vi "SessionName To IniTokenCluster.vi"(11 "trimmed string":string) -> (3 "IniTokenCluster":T1)   [LabVIEW 2012]
uses:
  Def-IniTokenCluster.ctl
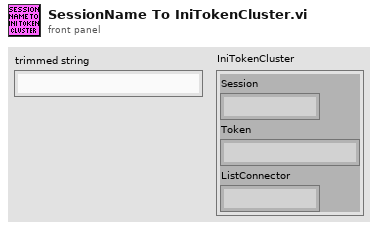
[diagram p1: front panel]
types:
  T1 = typedef "Def-IniTokenCluster.ctl" = cluster{"Session":string, "Token":string, "ListConnector":string}
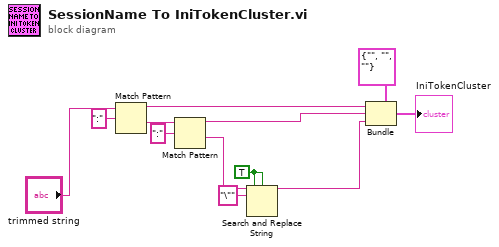
[diagram p0: block diagram]
diagram:
  w9 = TRUE ("ignore case? (F)")
  n1 = Match Pattern(string="trimmed string", regular expression=":") -> (before substring=w4:string, after substring=w1:string)  [unwired: 1 in, 2 out]
  n2 = Match Pattern(string=w1, regular expression=":") -> (before substring=w6:string, after substring=w7:string)  [unwired: 1 in, 2 out]
  n3 = Search and Replace String(replace all?=w9, case sensitive?=w9, input string=w7, search string="\"") -> (result string=w10:string)  [unwired: 4 in, 3 out]
  n4 = Bundle(cluster=T1 {"Session"="", "Token"="", "ListConnector"=""} ("IniTokenCluster"), "Session"=w4, "Token"=w6, "ListConnector"=w10) -> (→"IniTokenCluster":T1)
